vi "MGI Smooth 2D Array.vi"(1 "Array[][]":sgl[][](array[numeric]) format="%.2f") -> (0 "Smoothed Array[][]":sgl[][](array[numeric]) format="%.2f")   [LabVIEW 2020]
doc: "Perform a smoothing operation on a 2D array using a kernel like:\n0 1 0\n1 1 1\n0 1 0\nElement sums are normalized by the number of valid source elements, so a constant array would be unchanged.\n\nAuthored by David A. Moore\nsupport@mooregoodideas.com\nwww.mooregoodideas.com\n\nCopyright (c) 2010, Moore Good Ideas, Inc.\n\nAll rights reserved.\n\nRedistribution and use in source and binary forms, with or without modification, are permitted provided that the following conditions are met:\n\n * Redistributions of source code must retain the above copyright notice, this list of conditions and the following disclaimer.\n * Redistributions in binary form must reproduce the above copyright notice, this list of conditions and the following disclaimer in the documentation and/or other materials provided with the distribution.\n * Neither the name of Moore Good Ideas, Inc. nor the names of its contributors may be used to endorse or promote products derived from this software without specific prior written permission.\n\nTHIS SOFTWARE IS PROVIDED BY THE COPYRIGHT HOLDERS AND CONTRIBUTORS \"AS IS\" AND ANY EXPRESS OR IMPLIED WARRANTIES, INCLUDING, BUT NOT LIMITED TO, THE IMPLIED WARRANTIES OF MERCHANTABILITY AND FITNESS FOR A PARTICULAR PURPOSE ARE DISCLAIMED. IN NO EVENT SHALL THE COPYRIGHT OWNER OR CONTRIBUTORS BE LIABLE FOR ANY DIRECT, INDIRECT, INCIDENTAL, SPECIAL, EXEMPLARY, OR CONSEQUENTIAL DAMAGES (INCLUDING, BUT NOT LIMITED TO, PROCUREMENT OF SUBSTITUTE GOODS OR SERVICES; LOSS OF USE, DATA, OR PROFITS; OR BUSINESS INTERRUPTION) HOWEVER CAUSED AND ON ANY THEORY OF LIABILITY, WHETHER IN CONTRACT, STRICT LIABILITY, OR TORT (INCLUDING NEGLIGENCE OR OTHERWISE) ARISING IN ANY WAY OUT OF THE USE OF THIS SOFTWARE, EVEN IF ADVISED OF THE POSSIBILITY OF SUCH DAMAGE."
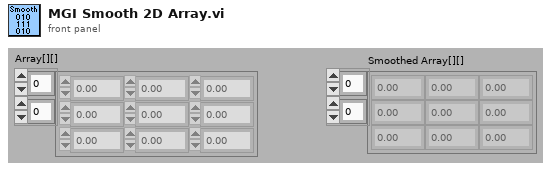
[diagram p1: front panel]
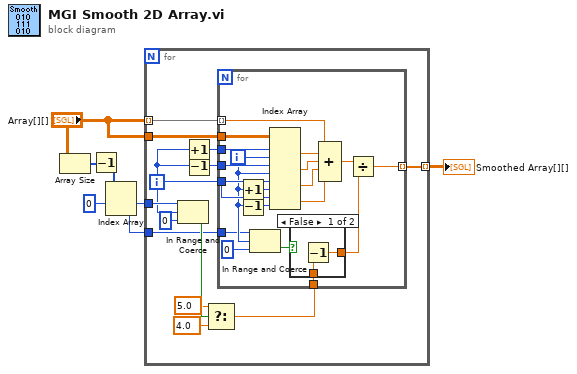
[diagram p0: block diagram]
diagram:
  n1 = Array Size(array="Array[][]") -> (size(s)=w6:i32[])
  n2 = Decrement(x=w6) -> (x-1=w3:i32[])
  n3 = Index Array(array=w3, index #1=0 ("index")) -> (element #1=w4:i32, element #2=w2:i32)  [unwired: 1 in]
  n4 = for {
    tunnel: "Array[][]" -> [w20] mode=indexing
    tunnel: "Array[][]" -> [w19]
    tunnel: w4 -> [w16]
    tunnel: w2 -> [w10]
    tunnel: [w8] -> w1 mode=indexing
    i -> [w15]
    n5 = In Range and Coerce(upper limit=w16, x=w15, lower limit=0) -> (In Range?=w13:bool)  [unwired: 1 out]
    n6 = Increment(x=w15) -> (x+1=w18:i32)
    n7 = Decrement(x=w15) -> (x-1=w17:i32)
    n8 = Select(t=sgl 5.0 ("lower limit"), s=w13, f=sgl 4.0) -> (s? t:f=w9:sgl)
    n9 = for {
      tunnel: w20 -> [w35] mode=indexing
      tunnel: w19 -> [w39]
      tunnel: w15 -> [w29]
      tunnel: w18 -> [w37]
      tunnel: w17 -> [w36]
      tunnel: w10 -> [w27]
      tunnel: w9 -> [w24]
      tunnel: [w21] -> w8 mode=indexing
      i -> [w28]
      n10 = Increment(x=w28) -> (x+1=w38:i32)
      n11 = Decrement(x=w28) -> (x-1=w30:i32)
      n12 = In Range and Coerce(upper limit=w27, x=w28, lower limit=0) -> (In Range?=w25:bool)  [unwired: 1 out]
      n13 = Index Array(array=w39, index (row) #1=w37, index (col) #1=w28, index (row) #2=w36, index (col) #2=w28, index (row) #3=w29, index (col) #3=w38, index (row) #4=w29, index (col) #4=w30) -> (element #1=w34:sgl, element #2=w33:sgl, element #3=w32:sgl, element #4=w31:sgl)
      n14 = case shown="False" w25 {
        tunnel: w24 -> [w41 w42]
        tunnel: [w40 w42] -> w22
        frame False {
          n15 = Decrement(x=w41) -> (x-1=w40:sgl)
        }
        frame True {
        }
      }
      n16 = Compound Arithmetic op=ADD(w35, w34, w33, w32, w31) -> (w23:sgl)
      n17 = Divide(x=w23, y=w22) -> (x/y=w21:sgl)
    }
  }
  "Smoothed Array[][]" <- w1
